vi "PH_Tektronix_7000.constructor.vi"(0 "name":string, 2 "data in":string, 5 "error in(no error)":errorcluster) -> (14 "i ref out":refnum<vi>, 16 "data out":string, 19 "error out":errorcluster)   [LabVIEW 2014, in "PH_Tektronix_7000.lvlib"]
doc: "This is the constructor of a class.\n\nLicense Agreement for this software:\n\nCopyright (C)\nGesellschaft für Schwerionenforschung, GSI\nPlanckstr. 1\n64291 Darmstadt\nGermany\n\nContact: D.Beck@gsi.de \n\nThis program is free software; you can redistribute it and/or modify it under the terms of the \nGNU General Public License as published by the Free Software Foundation; either version 2 of \nthe license, or (at your option) any later version.\n\nThis program is distributed in the hope that it will be useful, but WITHOUT ANY WARRANTY; \nwithout even the implied warranty of MERCHANTABILITY or FITNESS FOR A PARTICULAR PURPOSE. See the GNU General License for more details (http://www.gnu.org).\n\nGesellschaft für Schwerionenforschung, GSI\nPlanckstr. 1, 64291 Darmstadt, Germany\nFor all questions and ideas contact: M.Richter@gsi.de, H.Brand@gsi.de or D.Beck@gsi.de.\nLast update: 16-JUN-2004"
uses:
  PH_Tektronix_7000.lvlib
  CS_Core/CSSystem/CSSystemLib/CSSystemLib.lvlib
  PH_Basics/PH_PSDBWriter/PH_PSDBWriter.lvlib
  CS_Core/CSObj/CSObj.lvlib
  PH_Basics/PH_Class/PH_Class.lvlib
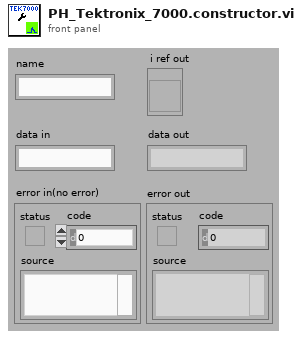
[diagram p1: front panel]
types:
  T1 = enum16{"SetAttribute", "GetAttribute", "CreateAttribute", "DestroyAttribute", "DestroyAllAtributes"}
  T2 = typedef "PH_Tektronix_7000.lvlib/PH_Tektronix_7000.i attribute.ctl" = cluster{"VISA Resource Name":refnum<visa-resource-name>, "IDN":cluster{"Instrument Driver":string, "Instrument Firmware":string, "Model":string, "Serial Number":string}, "Selftest":cluster{"Result":i32, "Message":string}, "Trigger Configuration":T3, "Acquisition Configuration":T4, "GUI Refs":T5, "State":T6, "Error Message":string, "Allow Prdc Loop?":bool, "Channel 1":T7, "Channel 2":T7, "Channel 3":T7, "Channel 4":T7, "Data CH 1":waveform(dbl), "Data CH 2":waveform(dbl), "Data CH 3":waveform(dbl), "Data CH 4":waveform(dbl), "Allow config?":bool, "Name Channel 1":string, "Name Channel 2":string, "Name Channel 3":string, "Name Channel 4":string, "Fetch Data before sending to PSDB?":bool, "Constructor passed?":bool, "Data taken at":timestamp, "Plot Colors":u32[], "Default VISA Resource":string}
  T3 = typedef "PH_Tektronix_7000.lvlib/PH_Tektronix_7000.Trigger Config.ctl" = cluster{"Source":u16, "Level [V]":dbl, "Slope":u16, "Coupling":u16, "Trigger Mode":u16}
  T4 = typedef "PH_Tektronix_7000.lvlib/PH_Tektronix_7000.Acquisition Config.ctl" = cluster{"Record Length":u32, "Timebase [s/div]":dbl, "Position [%]":dbl, "Acquisition Type":u16, "Average Waveforms":i32, "Envelope Waveforms":i32, "WfmDB Samples":i32, "Continuous?":bool, "Delay [s]":dbl, "Run?":bool}
  T5 = typedef "PH_Tektronix_7000.lvlib/PH_Tektronix_7000.GUI Refs.ctl" = cluster{"Graph":refnum<vi>, "State":refnum<vi>, "Delete":refnum<vi>, "VISA Resource":refnum<vi>, "Allow Configure":refnum<vi>, "Fetch Data":refnum<vi>, "Fetch before sending Data to PSDB":refnum<vi>, "Name Channel 1":refnum<vi>, "Name Channel 2":refnum<vi>, "Name Channel 3":refnum<vi>, "Name Channel 4":refnum<vi>, "Prdc Intervall [ms]":refnum<vi>, "Data taken":refnum<vi>, "Model":refnum<vi>, "Serial Number":refnum<vi>, "Firmware":refnum<vi>, "Driver":refnum<vi>, "Acquisition":refnum<vi>, "Trigger":refnum<vi>, "Cursor: D Time [s]":refnum<vi>, "Cursor: D Signal [V]":refnum<vi>, "Channel 1":refnum<vi>, "Channel 2":refnum<vi>, "Channel 3":refnum<vi>, "Channel 4":refnum<vi>}
  T6 = typedef "PH_StatusHandler.lvlib/PH_StatusHandler.Status.ctl" = i16
  T7 = typedef "PH_Tektronix_7000.lvlib/PH_Tektronix_7000.Channel Config.ctl" = cluster{"Enable Channel":bool, "Bandwidth":u16, "Input Impedance":u16, "Vertical Coupling":u16, "Probe Attenuation":dbl, "Range [V/div]":dbl, "Position [div]":dbl, "Bandwidth raw":string}
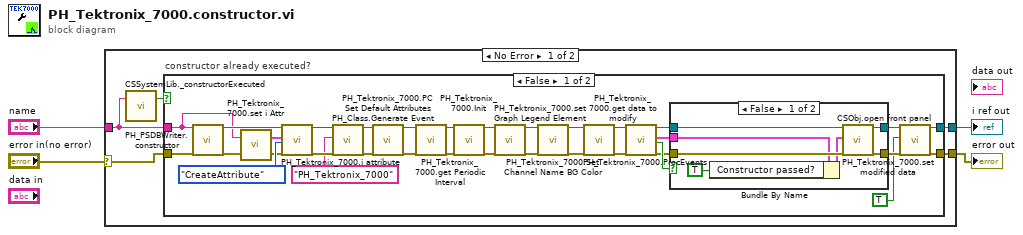
[diagram p0: block diagram]
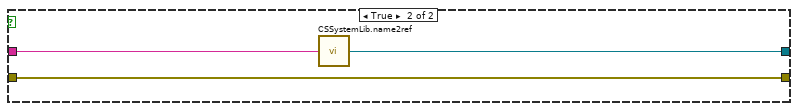
[diagram p3: hidden frame]
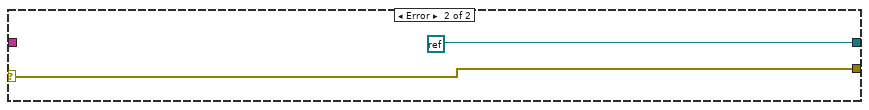
[diagram p4: hidden frame]
diagram:
  n1 = case shown="No Error" "error in(no error)" {
    selector: "error in(no error)" -> [w9 w55]
    tunnel: "name" -> [w8 _]
    tunnel: [w6 refnum<k0> refnum] -> w3
    tunnel: [w5 w55] -> w2
    frame No Error {
      n2 = call "CSSystemLib._constructorExecuted.vi"("name"=w8) -> ("constructor executed?"=w7:bool)  [unwired: 18 in]
      n3 = case "constructor already executed?" shown="False" w7 {
        tunnel: [w38 w53] -> w6
        tunnel: [w36 w52] -> w5
        tunnel: w9 -> [w14 w52]
        tunnel: w8 -> [w13 w54]
        frame False {
          n4 = call "PH_PSDBWriter.constructor.vi"("name"=w13, "error in"=w14) -> ("i ref out"=w21:refnum<vi>, "error out"=w12:errorcluster)  [unwired: 15 in, 1 out]
          n5 = call "PH_Tektronix_7000.set i Attr.vi"("error in (no error)"=w12, "DB Entry to read"=w13) -> ("error out"=w11:errorcluster, "i Attributes"=w10:T2)
          n6 = call "PH_Tektronix_7000.i attribute.vi"("VI Refnum"=w21, "CLASS.i attribute"=w10, "Action"=T1."CreateAttribute", "error in (no error)"=w11) -> ("VI Refnum out"=w19:refnum<vi>, "error out"=w17:errorcluster)  [unwired: 13 in, 1 out]
          n7 = call "PH_Class.Generate Event.vi"("i ref in"=w19, "Class"="PH_Tektronix_7000", "error in (no error)"=w17) -> ("i ref out"=w18:refnum<vi>, "error out"=w16:errorcluster)  [unwired: 15 in]
          n8 = call "PH_Tektronix_7000.PC Set Default Attributes.vi"("i ref in"=w18, "error in"=w16) -> ("i ref out"=w31:refnum<vi>, "error out"=w30:errorcluster)  [unwired: 16 in]
          n9 = call "PH_Tektronix_7000.get Periodic Interval.vi"("i ref in"=w31, "error in"=w30) -> ("i ref out"=w29:refnum<vi>, "error out"=w28:errorcluster)  [unwired: 16 in]
          n10 = call "PH_Tektronix_7000.Init.vi"("i ref in"=w29, "error in (no error)"=w28) -> ("i ref out"=w33:refnum<vi>, "error out"=w32:errorcluster)  [unwired: 16 in]
          n11 = call "PH_Tektronix_7000.set Graph Legend Element.vi"("i ref in"=w33, "error in (no error)"=w32) -> ("i ref out"=w26:refnum<vi>, "error out"=w27:errorcluster)  [unwired: 16 in]
          n12 = call "PH_Tektronix_7000.Set Channel Name BG Color.vi"("i ref in"=w26, "error in"=w27) -> ("i ref out"=w25:refnum<vi>, "error out"=w24:errorcluster)  [unwired: 16 in]
          n13 = call "PH_Tektronix_7000.ProcEvents.vi"("i ref in"=w25, "error in"=w24) -> ("i ref out"=w23:refnum<vi>, "error out"=w22:errorcluster)  [unwired: 16 in]
          n14 = call "PH_Tektronix_7000.get data to modify.vi"("i ref in"=w23, "error in (no error)"=w22) -> ("i ref out"=w42:refnum<vi>, "i attribute"=w41:T2, "timed out"=w40:bool, "error out"=w39:errorcluster)  [unwired: 14 in]
          n15 = case shown="False" w40 {
            tunnel: [w44 w51] -> w37
            tunnel: [w43 w50] -> w35
            tunnel: w39 -> [w49 w50]
            tunnel: w41 -> [w48 _]
            tunnel: w42 -> [w46 w51]
            frame False {
              n16 = Bundle By Name(cluster=w48, "Constructor passed?"=TRUE) -> (w47:T2)
              n17 = call "PH_Tektronix_7000.set modified data.vi"("i ref in"=w46, "i attribute"=w47, "error in (no error)"=w49) -> ("i ref out"=w44:refnum<vi>, "error out"=w43:errorcluster)  [unwired: 15 in]
            }
            frame True {
            }
          }
          n18 = call "CSObj.open front panel.vi"("i ref in"=w37, "frontPanelOpen"=TRUE, "error in (no error)"=w35) -> ("i ref out"=w38:refnum<vi>, "error out"=w36:errorcluster)  [unwired: 15 in]
        }
        frame True {
          n19 = call "CSSystemLib.name2ref.vi"("name"=w54) -> ("obj refnum"=w53:refnum<vi>)
        }
      }
    }
    frame Error {
    }
  }
  "i ref out" <- w3
  "error out" <- w2
